vi "Read Use Overdrive_.vi"(8 "error in (no error)":errorcluster, 11 "SemiProbe in":refnum<class "SemiProbe.lvclass">) -> (0 "error out":errorcluster, 2 "Use Overdrive?":bool, 3 "SemiProbe out":refnum<class "SemiProbe.lvclass">)   [LabVIEW 2018, in "SemiProbe.lvclass"]
uses:
  SemiProbe.lvclass
  SemiProbe.lvclass/SemiProbe.ctl
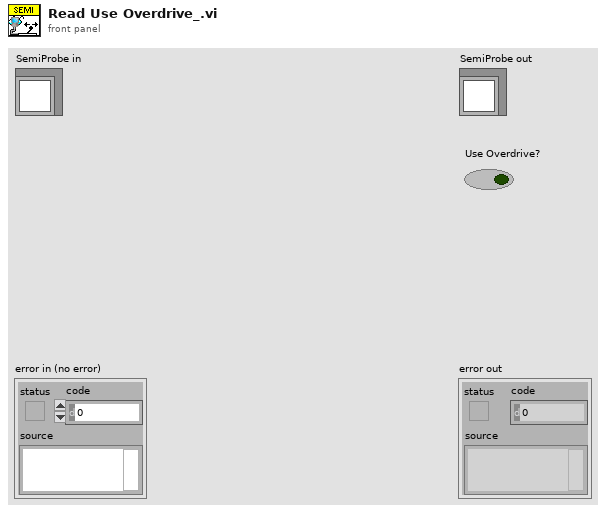
[diagram p1: front panel]
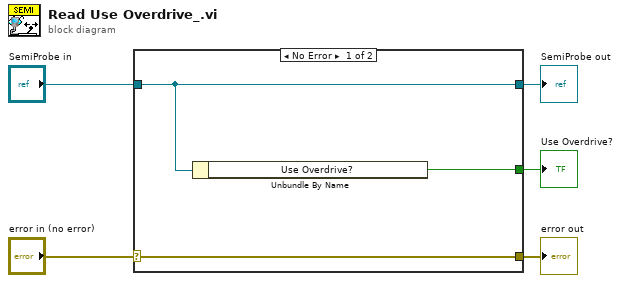
[diagram p0: block diagram]
diagram:
  n1 = case shown="No Error" "error in (no error)" {
    selector: "error in (no error)" -> [w8 w9]
    tunnel: [w8 w9] -> w4
    tunnel: [w7 w10] -> w2
    tunnel: "SemiProbe in" -> [w7 w10]
    tunnel: [w6 _] -> w1
    frame No Error {
      n2 = Unbundle By Name(w7) -> ("Use Overdrive?"=w6:bool)
    }
    frame Error {
    }
  }
  "error out" <- w4
  "SemiProbe out" <- w2
  "Use Overdrive?" <- w1
